vi "TreeNode Get Children.vi"(8 "error in (no error)":errorcluster, 11 "TreeNode DVR in":refnum<data-value>) -> (0 "error out":errorcluster, 1 "Children":i64[](array[numeric]), 3 "TreeNode DVR out":refnum<data-value>)   [LabVIEW 2012, in "MDSplus.lvlib"]
uses:
  <vilib>/MDSplus/Library/MDSplus.lvlib
  <vilib>/MDSplus/Classes/Data_Class/TreeNode_Class/TreeNode.lvclass
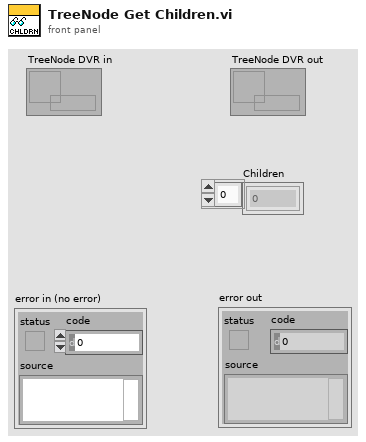
[diagram p1: front panel]
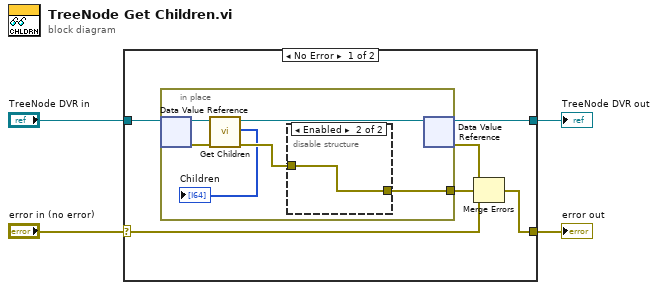
[diagram p0: block diagram]
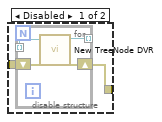
[diagram p2: hidden frame]
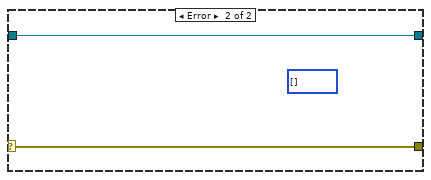
[diagram p3: hidden frame]
diagram:
  n1 = case shown="No Error" "error in (no error)" {
    selector: "error in (no error)" -> [w9 w25]
    tunnel: "TreeNode DVR in" -> [w10 w24]
    tunnel: [w6 w25] -> w4
    tunnel: [w7 w24] -> w1
    frame No Error {
      n2 = in-place {
        in-place-border: [w16] -> w5
        n3 = in-place-dvr #1(w10) -> (w15:refnum<class "TreeNode.lvclass">, w14:errorcluster)
        n4 = call-dynamic "Get Children.vi"("error in (no error)"=w14, "TreeNode in"=w15) -> ("error out"=w13:errorcluster, "Children"=→"Children":i64[], "TreeNode out"=w12:refnum<class "TreeNode.lvclass">)  [unwired: 7 in]
        n5 = disable-structure shown="Enabled" {
          disable-tunnel: [w18 w23] -> w16
          disable-tunnel: w13 -> [w17 w23]
          frame Disabled {
            n6 = for {
              tunnel: _ -> [w22] mode=indexing
              tunnel: [w21] -> _ mode=indexing
              shift-right: [w19] -> w18
              shift-left: w17 -> [w20]
              n7 = call <vilib>:"New TreeNode DVR.vi"("error in (no error)"=w20, "TreeNode in"=w22) -> ("error out"=w19:errorcluster, "TreeNode DVR out"=w21:refnum<data-value>)  [unwired: 8 in]
            }
          }
          frame Enabled {
          }
        }
        n8 = in-place-dvr #1(w12) -> (w7:refnum<data-value>, w8:errorcluster)
      }
      n9 = Merge Errors(w8, w5, w9) -> (w6:errorcluster)
    }
    frame Error {
      (unwired) i64[] [] ("Descendants")
    }
  }
  "error out" <- w4
  "TreeNode DVR out" <- w1
